vi "LEIN create custom return Q.vi"(11 "error in (no error)":errorcluster) -> (4 "LEIN custom reply Q":T1, 15 "error out":errorcluster)   [LabVIEW 2011]
uses:
  LEIN custom reply Q.ctl
  LEIN Reply Holder.ctl
  LEIN CMD Cluster.ctl
  LEIN CMD List.ctl
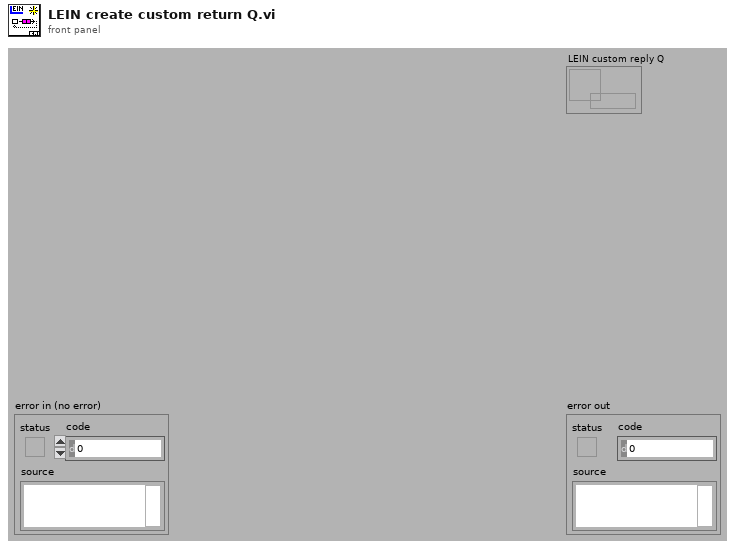
[diagram p1: front panel]
types:
  T1 = typedef "LEIN custom reply Q.ctl" = refnum<queue>
  T2 = typedef "LEIN Reply Holder.ctl" = cluster{"Reply msg(cmdif no reply)":T3, "Reply time":timestamp, "Valid reply":bool}
  T3 = typedef "LEIN CMD Cluster.ctl" = cluster{"SID":u8, "ANF":bool, "CMD":T4, "DATA":u8[]}
  T4 = typedef "LEIN CMD List.ctl" = enum8{"ACTI", "TASK", "RES0", "STAT", "RES1", "RES2", "RES3", "USER"}
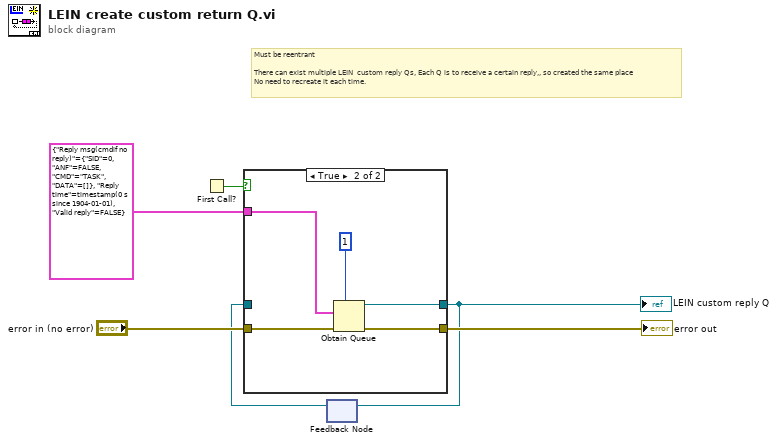
[diagram p0: block diagram]
diagram:
  # "Must be reentrant\n\nThere can exist multiple LEIN  custom reply Qs, Each Q is to receive a certain reply,, so created the same place\nNo need to recreate it each time."
  n1 = First Call?() -> (First Call?: T/F=w3:bool)
  n2 = feedback #1() -> (w1:refnum<queue>)  [unwired: 1 in]
  n3 = case shown="True" w3 {
    tunnel: T2 {"Reply msg(cmdif no reply)"={"SID"=0, "ANF"=FALSE, "CMD"=enum."TASK", "DATA"=[]}, "Reply time"=timestamp(0 s since 1904-01-01), "Valid reply"=FALSE} ("LEIN reply holder") -> [_ w13]
    tunnel: [w7 w11] -> w2
    tunnel: "error in (no error)" -> [w8 w10]
    tunnel: [w8 w9] -> w4
    tunnel: w1 -> [w7 _]
    frame False {
    }
    frame True {
      n4 = Obtain Queue(max queue size (-1, unlimited)=1, element data type=w13, error in (no error)=w10) -> (queue out=w11:refnum<queue>, error out=w9:errorcluster)  [unwired: 2 in, 1 out]
    }
  }
  "LEIN custom reply Q" <- w2
  "error out" <- w4
  n5 = feedback-in #1(w2) -> ()
